vi "__Alicat SD_ConfigRead.vi"(7 "error in (no error)":errorcluster) -> (0 "error out":errorcluster, 2 "AlicatsControl":T1=[["A", "SI", "398519", "N2", "100", "SLPM", "0.00", "0.00"], ["B", "SI", "398518", "N2", "100", "SLPM", "0.00", "0.00"], ["C", "SI", "428058", "Air", "100", "SLPM", "0.00", "0.00"], ["D", "NO", "--------", "------", "------", "------", "0.00", "0.00"]])   [LabVIEW 2017]
doc: "Illustrates how to create and write a configuration settings file.\n\nInstructions:\nEnter values in the controls on the front panel then click on the Run Arrow.\nTo read the file, run Read Configuration Settings File.vi located in the file\\config.llb."
uses:
  __s_TablaAlicats.ctl
  <vilib>/Utility/config.llb/Read Key (String).vi
  <vilib>/Utility/config.llb/NI_LVConfig.lvlib
panel:
  in  "?":bool
  out "configuration file path":path=path "C:/Users/criogenia/Documents/LabVIEW Data/AttoCube.ini"
  # "Instructions:\nEnter values in the controls below, then click on the Run arrow.  The VI will write\nthese values into the selected configuration settings file.\n\nTo read the file, run Read Configuration Settings File.vi located in the file\\config.llb."
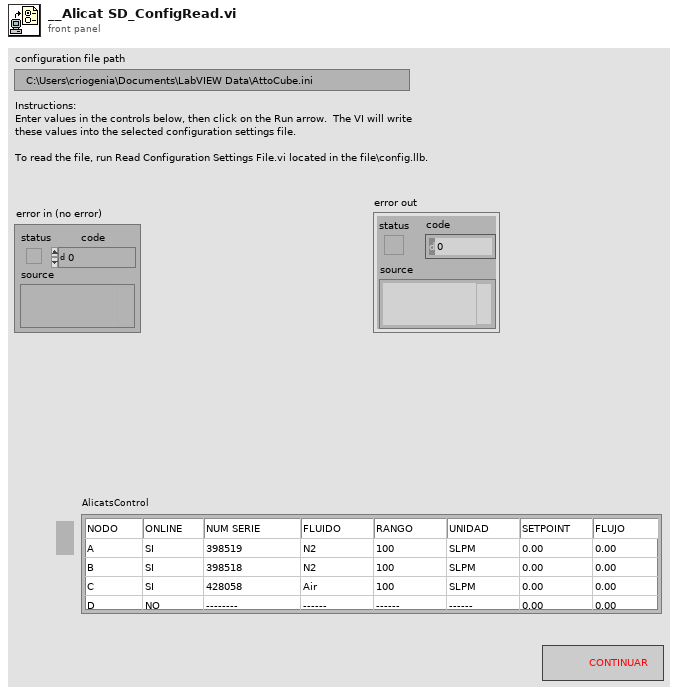
[diagram p1: front panel]
types:
  T1 = typedef "__s_TablaAlicats.ctl" = string[][]
  T2 = typedef "NI_LVConfig.lvlib/Config Data RefNum.ctl" = refnum<k1>
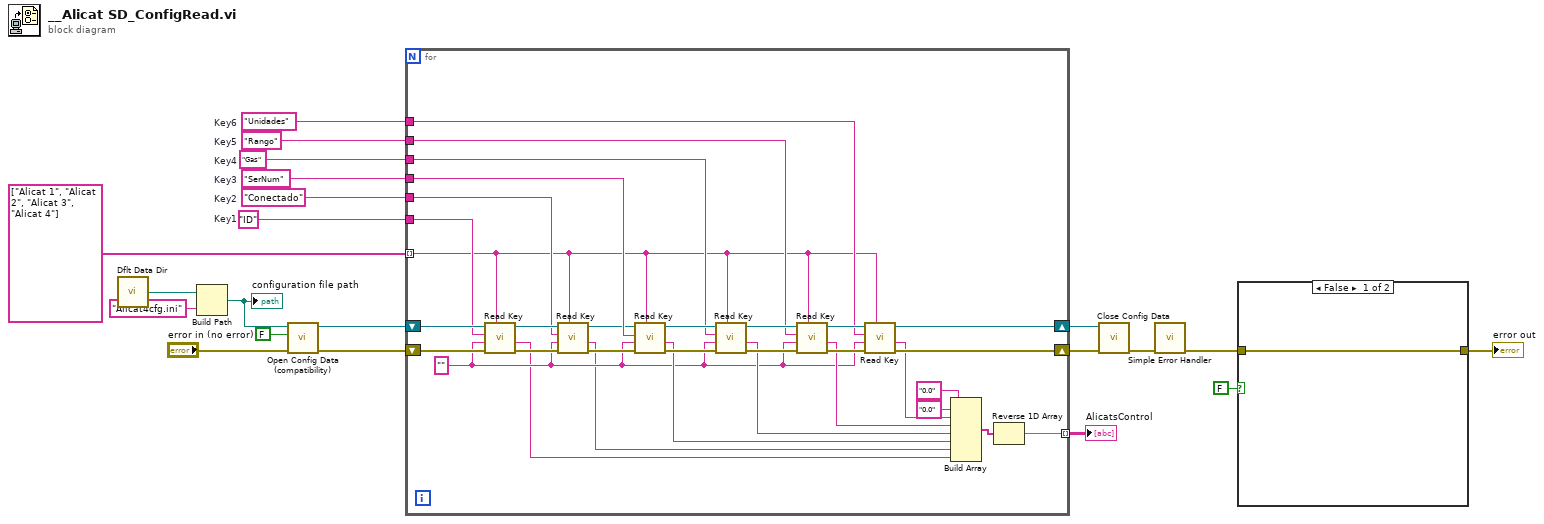
[diagram p0: block diagram]
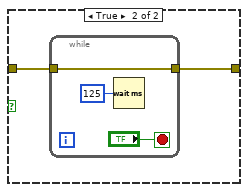
[diagram p2: hidden frame]
diagram:
  w2 = "Conectado"  # Key2
  w9 = "Unidades"  # Key6
  w11 = "Gas"  # Key4
  w10 = "Rango"  # Key5
  w12 = "SerNum"  # Key3
  w13 = "ID"  # Key1
  n1 = call <vilib>:"Dflt Data Dir.vi"() -> ("App:Default Data Directory"=w17:path)
  n2 = Build Path(base path=w17, name or relative path="Alicat4cfg.ini") -> (appended path=w16:path)
  "configuration file path" <- w16
  n3 = call <vilib>:"Open Config Data (compatibility).vi"("error in (no error)"="error in (no error)", "create file if necessary (T)"=FALSE ("create file if necessary? (T)"), "configuration file path"=w16) -> ("error out"=w20:errorcluster, "refnum"=w21:T2)  [unwired: 6 in, 1 out]
  n4 = for {
    tunnel: string[] ["Alicat 1", "Alicat 2", "Alicat 3", "Alicat 4"] -> [w27] mode=indexing
    tunnel: w13 -> [w45]
    tunnel: w12 -> [w44]
    tunnel: w11 -> [w43]
    tunnel: w10 -> [w42]
    tunnel: w9 -> [w41]
    shift-right: [w39] -> w6
    shift-left: w21 -> [w53]
    shift-right: [w40] -> w5
    shift-left: w20 -> [w52]
    tunnel: [w33] -> w7 mode=indexing
    tunnel: w2 -> [w28]
    w26 = ""
    n5 = call-poly <vilib>:"Read Key.vi"("section"=w27, "error in (no error)"=w52, "default value"=w26, "key"=w45, "refnum"=w53) -> ("error out"=w30:errorcluster, "value"=w25:string, "refnum out"=w32:T2)  [unwired: 3 in, 1 out]
    n6 = call-poly <vilib>:"Read Key.vi"("section"=w27, "error in (no error)"=w30, "default value"=w26, "key"=w28, "refnum"=w32) -> ("error out"=w29:errorcluster, "value"=w24:string, "refnum out"=w31:T2)  [unwired: 3 in, 1 out]
    n7 = call-poly <vilib>:"Read Key.vi"("section"=w27, "error in (no error)"=w29, "default value"=w26, "key"=w44, "refnum"=w31) -> ("error out"=w50:errorcluster, "value"=w35:string, "refnum out"=w51:T2)  [unwired: 3 in, 1 out]
    n8 = call-poly <vilib>:"Read Key.vi"("section"=w27, "error in (no error)"=w50, "default value"=w26, "key"=w43, "refnum"=w51) -> ("error out"=w49:errorcluster, "value"=w36:string, "refnum out"=w48:T2)  [unwired: 3 in, 1 out]
    n9 = call-poly <vilib>:"Read Key.vi"("section"=w27, "error in (no error)"=w49, "default value"=w26, "key"=w42, "refnum"=w48) -> ("error out"=w47:errorcluster, "value"=w37:string, "refnum out"=w46:T2)  [unwired: 3 in, 1 out]
    n10 = call-poly <vilib>:"Read Key.vi"("section"=w27, "error in (no error)"=w47, "default value"=w26, "key"=w41, "refnum"=w46) -> ("error out"=w40:errorcluster, "value"=w38:string, "refnum out"=w39:T2)  [unwired: 3 in, 1 out]
    n11 = Build Array("0.0" ("element"), "0.0" ("element"), w38, w37, w36, w35, w24, w25) -> (w34:string[])
    n12 = Reverse 1D Array(array=w34) -> (reversed array=w33:string[])
  }
  "AlicatsControl" <- w7
  n13 = call <vilib>:"Close Config Data.vi"("error in (no error)"=w5, "refnum"=w6) -> ("error out"=w8:errorcluster)  [unwired: 8 in, 1 out]
  n14 = call <vilib>:"Simple Error Handler.vi"("error in (no error)"=w8) -> ("error out"=w4:errorcluster)  [unwired: 4 in, 4 out]
  n15 = case shown="False" FALSE {
    tunnel: w4 -> [w54 w56]
    tunnel: [w54 w55] -> w3
    frame False {
    }
    frame True {
      n16 = while {
        tunnel: w56 -> [w58]
        tunnel: [w58] -> w55
        stop <- "?" stop-if-true
        n17 = Wait (ms)(milliseconds to wait=u32 125) -> ()  [unwired: 1 out]
      }
    }
  }
  "error out" <- w3
